vi "Get Attributes.vi"(5 "Flatten Pointer?":bool, 7 "Test ID":string, 8 "error in (no error)":errorcluster, 10 "Include Private?":bool, 11 "Test Executive Ref":refnum<data-value>) -> (0 "error out":errorcluster, 1 "Attributes":variant[](array[variant]), 2 "Attribute Names out":string[](array[string]), 3 "Test Executive Ref out":refnum<data-value>, 4 "Data IDs":string[](array[string]), 6 "Found?":bool)   [LabVIEW 2020, in "Test Executive.lvlib" / "TestExecutive Ref.lvclass"]
uses:
  <vilib>/gpm_packages/@cs/test-executive/Source/Test Executive/TestExecutive Ref/TestExecutive Ref.lvclass
  <vilib>/gpm_packages/@cs/test-executive/Source/Test Executive/ITestExecutive/ITest Executive.lvclass
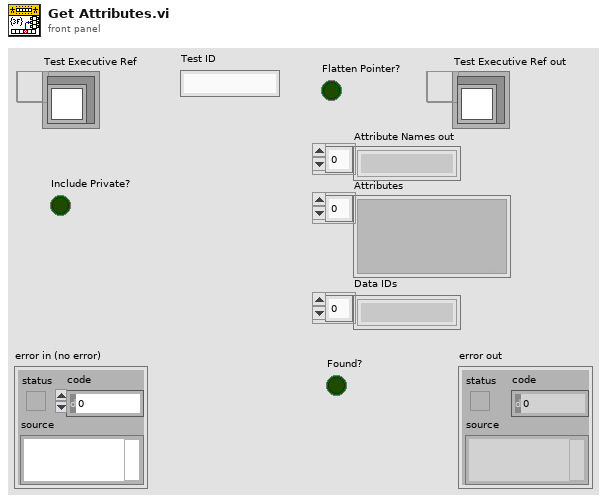
[diagram p1: front panel]
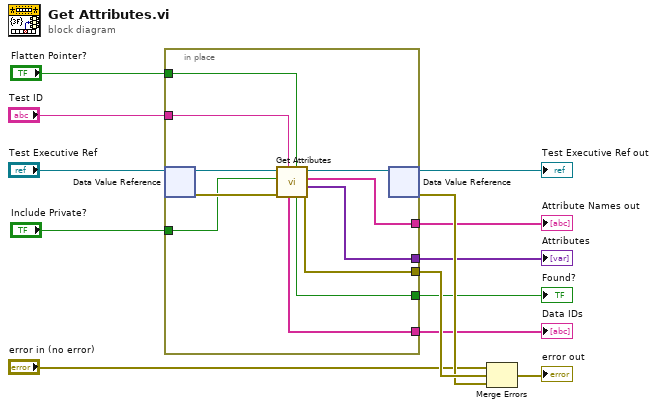
[diagram p0: block diagram]
diagram:
  n1 = in-place {
    in-place-border: [w23] -> w13
    in-place-border: "Test ID" -> [w20]
    in-place-border: "Flatten Pointer?" -> [w19]
    in-place-border: "Include Private?" -> [w18]
    in-place-border: [w17] -> w4
    in-place-border: [w16] -> w3
    in-place-border: [w15] -> w2
    in-place-border: [w14] -> w1
    n2 = in-place-dvr #1("Test Executive Ref") -> (w22:refnum<class "ITest Executive.lvclass">, w24:errorcluster)
    n3 = call-dynamic "Get Attributes.vi"("Flatten Pointer?"=w19, "Test ID"=w20, "error in (no error)"=w24, "Include Private?"=w18, "ITest Executive in"=w22) -> ("error out"=w23:errorcluster, "Attributes"=w16:variant[], "Attribute Names out"=w17:string[], "ITest Executive out"=w21:refnum<class "ITest Executive.lvclass">, "Found?"=w15:bool, "Data IDs"=w14:string[])  [unwired: 1 in]
    n4 = in-place-dvr #1(w21) -> (→"Test Executive Ref out":refnum<data-value>, w12:errorcluster)
  }
  "Attribute Names out" <- w4
  "Attributes" <- w3
  "Found?" <- w2
  "Data IDs" <- w1
  n5 = Merge Errors("error in (no error)", w13, w12) -> (→"error out":errorcluster)
